vi "_Get Server Control.vi"(4 "error in (no error)":errorcluster, 6 "Control Name":string, 7 "All Controls[]":refnum<vi>[](array[refnum])) -> (0 "error out":errorcluster, 2 "Ctl Refnum":refnum<vi>, 3 "All Controls[] out":refnum<vi>[](array[refnum]))   [LabVIEW 2012]
panel:
  # "It takes normally 1-5 ms to complete"
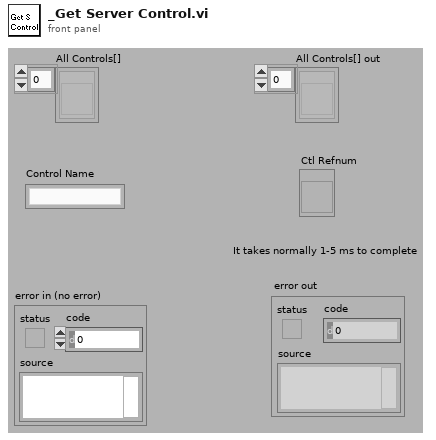
[diagram p1: front panel]
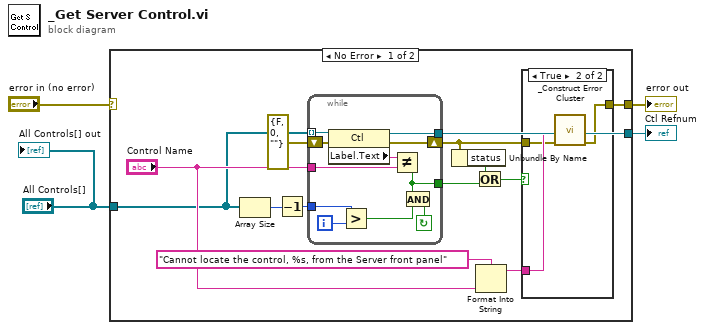
[diagram p0: block diagram]
diagram:
  n1 = case shown="No Error" "error in (no error)" {
    selector: "error in (no error)" -> [_ w32]
    tunnel: [w17 _] -> w4
    tunnel: [w16 w32] -> w3
    tunnel: "All Controls[]" -> [w6 _]
    frame No Error {
      n2 = Array Size(array=w6) -> (size(s)=w13:i32)
      n3 = Decrement(x=w13) -> (x-1=w12:i32)
      n4 = while {
        tunnel: w6 -> [w31] mode=indexing
        tunnel: w12 -> [w29]
        tunnel: "Control Name" -> [w27]
        tunnel: [w24] -> w17
        shift-right: [w22] -> w9
        shift-left: errorcluster {"status"=FALSE, "code"=0, "source"=""} ("error out") -> [w23]
        tunnel: [w21] -> w15
        i -> [w30]
        stop <- w26 continue-if-true
        n5 = property class="Ctl"(reference=w31, error in=w23) -> (reference out=w24:refnum<vi>, error out=w22:errorcluster, "Label.Text"=w28:string)
        n6 = Greater?(x=w29, y=w30) -> (0:w25:bool)
        n7 = Not Equal?(x=w28, y=w27) -> (x != y?=w21:bool)
        n8 = And(x=w21, y=w25) -> (x .and. y?=w26:bool)
      }
      n9 = Unbundle By Name(w9) -> ("status"=w14:bool)
      n10 = Or(x=w14, y=w15) -> (x .or. y?=w8:bool)
      n11 = Format Into String(format string="Cannot locate the control, %s, from the Server front panel", "Control Name") -> (resulting string=w10:string)  [unwired: 2 in, 1 out]
      n12 = case shown="True" w8 {
        tunnel: w10 -> [_ w20]
        tunnel: w9 -> [_ w19]
        tunnel: [_ w18] -> w16
        frame False {
        }
        frame True {
          n13 = call "_Construct Error Cluster.vi"("error in"=w19, "reason"=w20) -> ("error out"=w18:errorcluster)  [unwired: 2 in, 3 out]
        }
      }
    }
    frame Error {
    }
  }
  "error out" <- w3
  "Ctl Refnum" <- w4
  "All Controls[] out" <- "All Controls[]"
